vi "test_niScope.vi"() -> ()   [LabVIEW 2020, in "niScope Virtual Digitizer.lvlib"]
uses:
  niScope Virtual Digitizer.lvlib
  niScope Session.ctl
  niScope Virtual Channel Config.ctl
  niScope Virtual Channel Mode.ctl
  niScope Virtual Channel Input Z.ctl
  niScope Virtual Channel Coupling.ctl
  niScope Type.ctl
  niScope Digitizing Process Options.ctl
  niScope Data Packet.ctl
  niScope Trigger Setup.ctl
  <instrlib>/niScope/Controls/niScope trigger coupling.ctl
  <instrlib>/niScope/Controls/niScope trigger slope.ctl
  niScope Reference Clock.ctl
panel:
  in  "btn stop":bool
  out "offset [smpl]":i32
  out "temp [deg C]":dbl[][](graph)
  in  "decimate by":i32=10000
  out "sampling?":bool
  out "queue buffer [%]":dbl format="%1.1f"
  in  "use streaming":bool
  in  "channels":T1[](array[typedef]) {"Range [Vpk]" min=0.0; "Channel" min=0}
  out "card buffer [%]":dbl format="%1.1f"
  out "size(s)":i32[](array[numeric])
  out "Waveform Graph":dbl[][](graph)
  in  "samples count":i32=50000 min=1 format="%.0p"
  in  "fs [Hz]":dbl=50000.0 format="%#_6p"
  out "error out":errorcluster
  out "combined idn string":string
  in  "btn start":bool
  in  "niScope":T5={"channel cfg"=[], "sessions"=[], "multi cards"=FALSE, "channels"=0, "type"=enum."n/a", "memory [B/chn]"=0, "ext. clock [Hz]"=0.0, "samples count"=0, "use streaming"=FALSE, "proc setup"={"packet size [smpl]"=0, "current timeout [s]"=0.0, "blk2blk timeout [s]"=0.0, "event time"=timestamp(0 s since 1904-01-01), "temp sampl T [s]"=0.0, "data queue"=refnum, "stop notifier"=refnum, "proc ref"=refnum}, "sample width [B]"=0, "ranges [V]"=[], "trigger setup"={"coupling"=1, "level [V]"=0.0, "slope"=0, "mode"=enum."Immediate"}, "fs [Hz]"=0.0, "bitres [bit]"=0, "clock source"=enum."VAL_NO_SOURCE"} {"trigger setup"."level [V]" format="%.2f"; "trigger setup"."coupling" items=["AC"=0, "DC"=1, "HF Reject"=3, "LF Reject"=4, "AC Plus HF Reject"=1001]; "channel cfg"."Range [Vpk]" min=0.0; "channel cfg"."Channel" min=0}
  in  "btn exit":bool
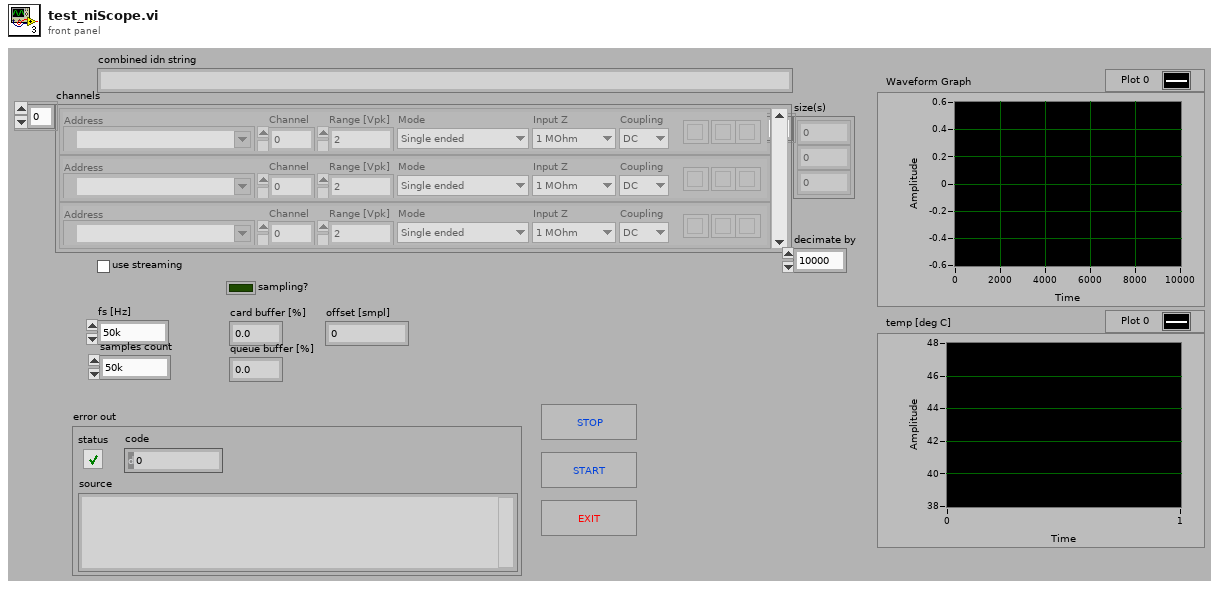
[diagram p1: front panel]
types:
  T1 = typedef "niScope Virtual Digitizer.lvlib/niScope Virtual Channel Config.ctl" = cluster{"Address":refnum<k15>, "Channel":i32, "Mode":T2, "Input Z":T3, "Coupling":T4, "Range [Vpk]":dbl, "btn clr":bool, "btn up":bool, "btn down":bool}
  T2 = typedef "niScope Virtual Digitizer.lvlib/niScope Virtual Channel Mode.ctl" = enum16{"Single ended", "Unbal. differential", "Differential"}
  T3 = typedef "niScope Virtual Digitizer.lvlib/niScope Virtual Channel Input Z.ctl" = enum16{"1 MOhm", "50 Ohm"}
  T4 = typedef "niScope Virtual Digitizer.lvlib/niScope Virtual Channel Coupling.ctl" = enum16{"AC", "DC", "GND"}
  T5 = typedef "niScope Virtual Digitizer.lvlib/niScope Session.ctl" = cluster{"channel cfg":T1[], "sessions":refnum<k20>[], "multi cards":bool, "channels":i32, "type":T6, "memory [B/chn]":i32, "ext. clock [Hz]":dbl, "samples count":i64, "use streaming":bool, "proc setup":T7, "sample width [B]":i32, "ranges [V]":dbl[], "trigger setup":T8, "fs [Hz]":dbl, "bitres [bit]":i32, "clock source":T11}
  T6 = typedef "niScope Virtual Digitizer.lvlib/niScope Type.ctl" = enum16{"n/a", "5922"}
  T7 = typedef "niScope Virtual Digitizer.lvlib/niScope Digitizing Process Options.ctl" = cluster{"packet size [smpl]":i64, "current timeout [s]":dbl, "blk2blk timeout [s]":dbl, "event time":timestamp, "temp sampl T [s]":dbl, "data queue":refnum<queue>, "stop notifier":refnum<notifier>, "proc ref":refnum<vi>}
  T8 = typedef "niScope Virtual Digitizer.lvlib/niScope Trigger Setup.ctl" = cluster{"coupling":T9, "level [V]":dbl, "slope":T10, "mode":enum16{"Immediate", "External", "Level"}}
  T9 = typedef "niScope trigger coupling.ctl" = u16
  T10 = typedef "niScope trigger slope.ctl" = i32
  T11 = typedef "niScope Virtual Digitizer.lvlib/niScope Reference Clock.ctl" = enum16{"VAL_NO_SOURCE", "VAL_CLK_IN", "VAL_PXI_CLOCK", "VAL_EXTERNAL"}
  T12 = typedef "niScope Virtual Digitizer.lvlib/niScope Record Aux Data.ctl" = cluster{"T smpl":i64[], "T [deg C]":dbl[][], "time stamp [s]":dbl[], "offset":dbl[], "gain":dbl[], "increment [s]":dbl, "valid?":bool, "abs timestamp":timestamp}
  T13 = typedef "niScope Virtual Digitizer.lvlib/niScope Data Packet.ctl" = cluster{"int32":i32[][], "card buffer [%]":dbl, "all done?":bool, "offset [smpl]":i64, "sampling?":bool, "queue buffer [%]":dbl, "int16":i16[][], "is int16?":bool, "count [smpl]":i32, "valid?":bool}
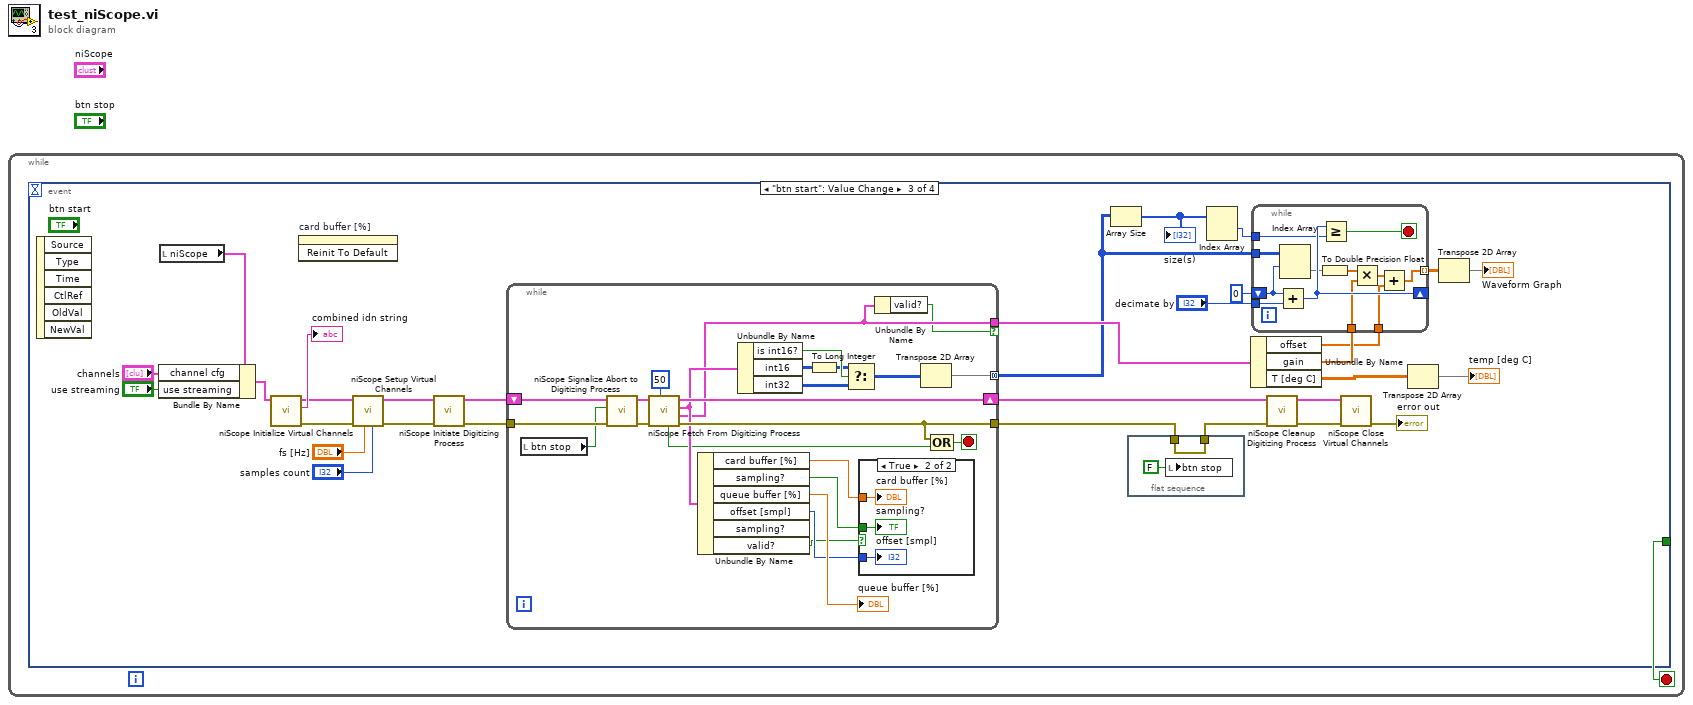
[diagram p0: block diagram]
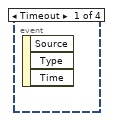
[diagram p2: hidden frame]
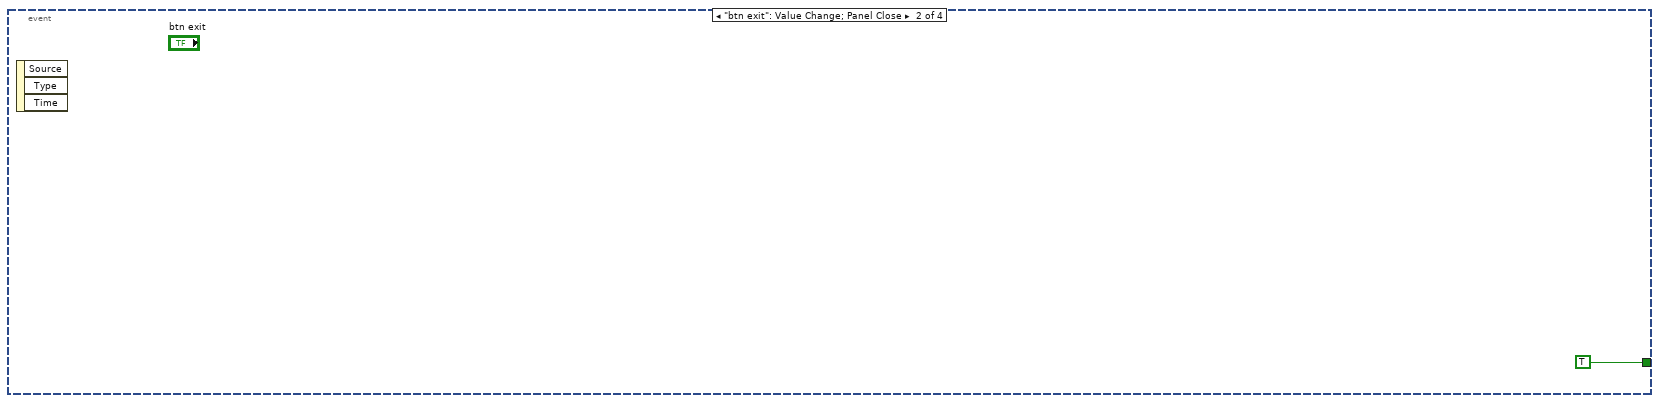
[diagram p3: hidden frame]
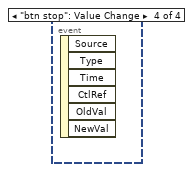
[diagram p5: hidden frame]
diagram:
  n1 = while {
    stop <- w1 stop-if-true
    n2 = event shown="[2] \"btn start\": Value Change" {
      selector: _ -> [_ _ _ _]
      dyn-events: _ -> [_ _ _ _]
      timeout: _ -> [_ _ _ _]
      tunnel: [_ TRUE _ _] -> w1
      event Timeout {
        n3 = event-data() -> ()  [unwired: 1 in, 3 out]
      }
      event "btn exit": Value Change; Panel Close {
        n4 = event-data() -> ()  [unwired: 1 in, 3 out]
      }
      event "btn start": Value Change {
        n5 = event-data() -> ()  [unwired: 1 in, 6 out]
        n6 = local read "niScope"() -> (w14:T5)
        n7 = Bundle By Name(cluster=w14, "channel cfg"="channels", "use streaming"="use streaming") -> (w15:T5)
        n8 = call "niScope Initialize Virtual Channels.vi"("niScope in"=w15) -> ("error out"=w31:errorcluster, "combined idn string"=→"combined idn string":string, "niScope out"=w30:T5)  [unwired: 7 in, 1 out]
        n9 = invoke on="card buffer [%]" class="DigNum (strict)" method="Reinit To Default"() -> ()  [unwired: 3 in, 3 out]
        n10 = call "niScope Setup Virtual Channels.vi"("samples count"="samples count", "fs [Hz]"="fs [Hz]", "error in"=w31, "niScope in"=w30) -> ("error out"=w27:errorcluster, "niScope out"=w26:T5)  [unwired: 6 in]
        n11 = call "niScope Initiate Digitizing Process.vi"("error in"=w27, "niScope in"=w26) -> ("error out"=w25:errorcluster, "niScope out"=w21:T5)  [unwired: 8 in]
        n12 = while {
          tunnel: w25 -> [w49]
          tunnel: [w57] -> w4
          tunnel: [w55] -> w7 mode=concatenating
          tunnel: [w44] -> w11 if=w43
          shift-right: [w59] -> w22
          shift-left: w21 -> [w48]
          stop <- w56 stop-if-true
          n13 = local read "btn stop"() -> (w45:bool)
          n14 = call "niScope Signalize Abort to Digitizing Process.vi"("error in"=w49, "send abort signal? (True)"=w45, "niScope in"=w48) -> ("error out (copy)"=w47:errorcluster, "niScope out (copy)"=w46:T5)  [unwired: 7 in]
          n15 = call "niScope Fetch From Digitizing Process.vi"("max wait for packet [ms]"=50, "error in"=w47, "niScope in"=w46) -> ("error out"=w57:errorcluster, "auxiliary sampling data"=w44:T12, "data block"=w51:T13, "niScope out"=w59:T5, "fetching done?"=w42:bool)  [unwired: 4 in]
          n16 = Unbundle By Name(w51) -> ("card buffer [%]"=w54:dbl, "sampling?"=w52:bool, "queue buffer [%]"=→"queue buffer [%]":dbl, "offset [smpl]"=w50:i64, "valid?"=w41:bool)  [unwired: 1 out]
          n17 = Unbundle By Name(w51) -> ("is int16?"=w40:bool, "int16"=w39:i16[][], "int32"=w38:i32[][])
          n18 = To Long Integer(number=w39) -> (32bit integer=w37:i32[][])
          n19 = Select(t=w37, s=w40, f=w38) -> (s? t:f=w36:i32[][])
          n20 = case shown="True" w41 {
            tunnel: w54 -> [_ w62]
            tunnel: w52 -> [_ w61]
            tunnel: w50 -> [_ w60]
            frame False {
            }
            frame True {
              "card buffer [%]" <- w62
              "sampling?" <- w61
              "offset [smpl]" <- w60
            }
          }
          n21 = Unbundle By Name(w44) -> ("valid?"=w43:bool)
          n22 = Transpose 2D Array(2D array=w36) -> (transposed array=w55:i32[][])
          n23 = Compound Arithmetic op=OR(w57, w42) -> (w56:bool)
        }
        n24 = Array Size(array=w7) -> (size(s)=w20:i32[])
        "size(s)" <- w20
        n25 = flat-sequence {
          tunnel: [w34] -> w3
          tunnel: w4 -> [w34]
          frame #0 {
            n26 = local write "btn stop"(FALSE ("btn stop")) -> ()
          }
        }
        n27 = Index Array(array=w20) -> (element #1=w16:i32)  [unwired: 2 in, 1 out]
        n28 = Unbundle By Name(w11) -> ("offset"=w9:dbl[], "gain"=w10:dbl[], "T [deg C]"=w6:dbl[][])
        n29 = while {
          tunnel: w16 -> [w71]
          tunnel: w7 -> [w74]
          shift-right: [w72] -> _
          shift-left: 0 -> [w69]
          tunnel: [w63] -> w17 mode=indexing
          tunnel: "decimate by" -> [w73]
          tunnel: w10 -> [w66]
          tunnel: w9 -> [w64]
          stop <- w70 stop-if-true
          n30 = Add(x=w69, y=w73) -> (x+y=w72:i32)
          n31 = Index Array(array=w74, index (row)=w69) -> (element=w68:i32[])  [unwired: 1 in]
          n32 = To Double Precision Float(number=w68) -> (double precision float=w67:dbl[])
          n33 = Greater Or Equal?(x=w72, y=w71) -> (x >= y?=w70:bool)
          n34 = Multiply(x=w67, y=w66) -> (x*y=w65:dbl[])
          n35 = Add(x=w65, y=w64) -> (x+y=w63:dbl[])
        }
        n36 = call "niScope Cleanup Digitizing Process.vi"("error in"=w3, "niScope in"=w22) -> ("error out"=w24:errorcluster, "niScope out"=w23:T5)  [unwired: 8 in]
        n37 = call "niScope Close Virtual Channels.vi"("error in"=w24, "niScope in"=w23) -> ("error out"=→"error out":errorcluster)  [unwired: 8 in, 1 out]
        n38 = Transpose 2D Array(2D array=w6) -> (transposed array=→"temp [deg C]":dbl[][])
        n39 = Transpose 2D Array(2D array=w17) -> (transposed array=→"Waveform Graph":dbl[][])
      }
      event "btn stop": Value Change {
        n40 = event-data() -> ()  [unwired: 1 in, 6 out]
      }
    }
  }
